vi "get transition voltages.vi"(7 "# of Samples":i32=5, 9 "Enum":enum16{"Ignite", "Quench"}(ring), 10 "Diode":tag, 11 "Main RF":tag) -> (1 "mean":dbl format="%0.2f")   [LabVIEW 2018]
uses:
  <vilib>/DAQmx/write.llb/DAQmx Write (Analog DBL 1Chan 1Samp).vi
  d16da458-7398-4570-a4bb-f738f0a42735.vi
  <vilib>/DAQmx/read.llb/DAQmx Read (Analog DBL 1Chan 1Samp).vi
  <vilib>/DAQmx/create/channels.llb/DAQmx Create Channel (AI-Voltage-Basic).vi
  <vilib>/DAQmx/create/channels.llb/DAQmx Create Channel (AO-Voltage-Basic).vi
  <vilib>/DAQmx/miscellaneous.llb/DAQmx Fill In Error Info.vi
  <vilib>/Analysis/NI_AALBase.lvlib
panel:
  out "Current Diode Voltage":dbl format="%0.2f"
  in  "Slow Factor":dbl=1.0
  out "Threshold":dbl
  out "Waveform Chart":dbl(graph)
  out "Current VO":dbl
  out "Previous Transition Voltage":dbl
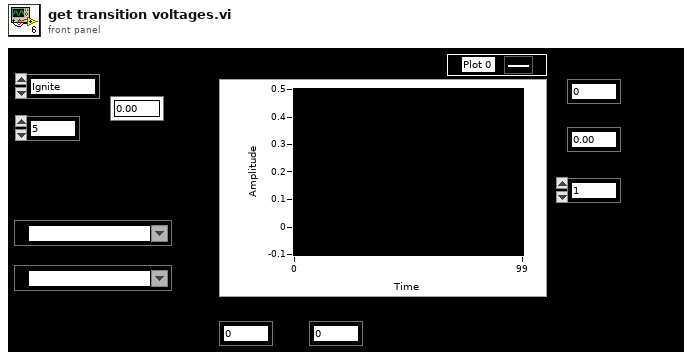
[diagram p1: front panel]
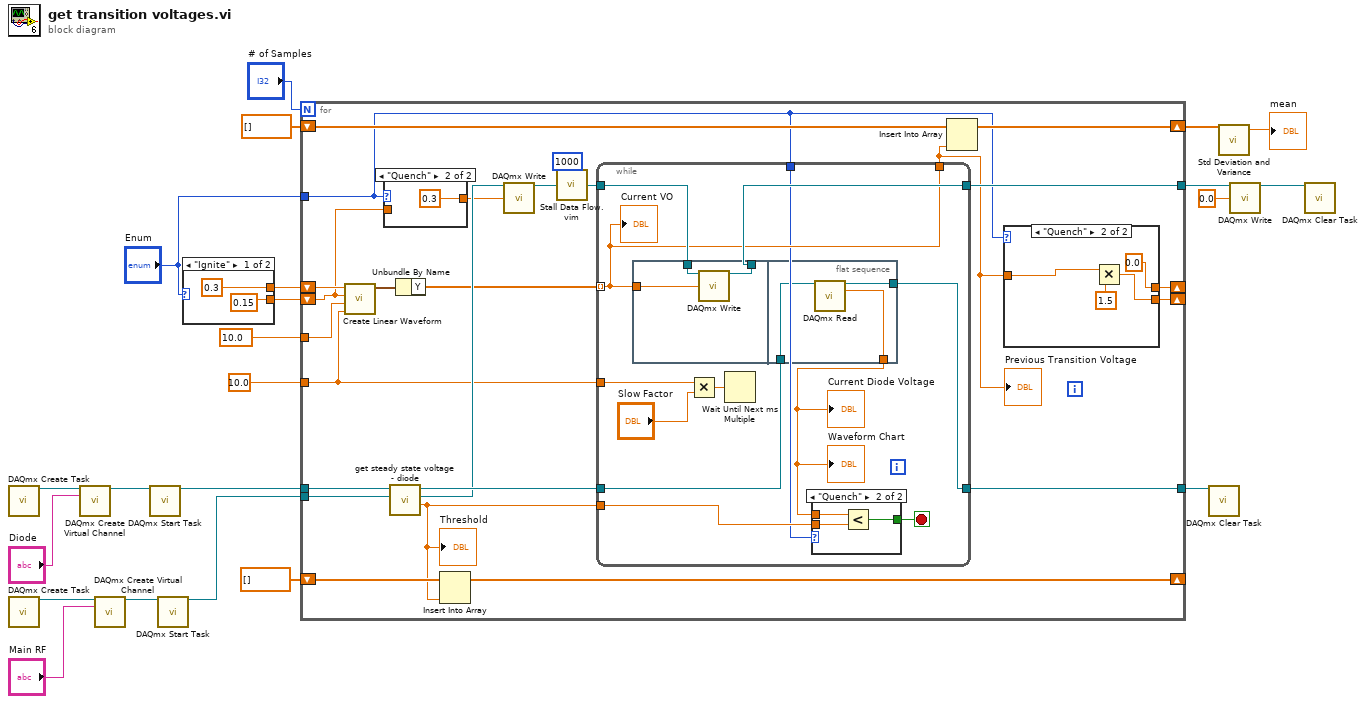
[diagram p0: block diagram]
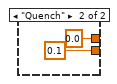
[diagram p2: hidden frame]
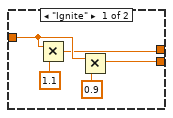
[diagram p3: hidden frame]
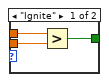
[diagram p5: hidden frame]
diagram:
  n1 = call <vilib>:"DAQmx Create Task.vi"() -> ("task out"=w21:refnum<k21>)  [unwired: 14 in, 1 out]
  n2 = call <vilib>:"DAQmx Create Task.vi"() -> ("task out"=w19:refnum<k21>)  [unwired: 14 in, 1 out]
  n3 = call-poly <vilib>:"DAQmx Create Virtual Channel.vi"("task in"=w21, "physical channels"="Diode") -> ("task out"=w15:refnum<k21>)  [unwired: 12 in, 1 out]
  n4 = call-poly <vilib>:"DAQmx Create Virtual Channel.vi"("task in"=w19, "physical channels"="Main RF") -> ("task out"=w14:refnum<k21>)  [unwired: 12 in, 1 out]
  n5 = call <vilib>:"DAQmx Start Task.vi"("task/channels in"=w15) -> ("task out"=w11:refnum<k21>)  [unwired: 13 in, 1 out]
  n6 = call <vilib>:"DAQmx Start Task.vi"("task/channels in"=w14) -> ("task out"=w10:refnum<k21>)  [unwired: 13 in, 1 out]
  n7 = case shown="\"Ignite\"" "Enum" {
    tunnel: [0.3 ("Vmax") 0.0 ("Vmax")] -> w9
    tunnel: [0.15 ("Vmin") 0.1 ("Vmin")] -> w8
    frame "Ignite" {
    }
    frame "Quench" {
    }
  }
  n8 = for {
    N: "# of Samples" -> [_]
    tunnel: w10 -> [w49]
    tunnel: [w36] -> w17
    tunnel: w11 -> [w50]
    tunnel: 10.0 ("Period") -> [w47]
    tunnel: 10.0 ("dt") -> [w46]
    shift-right: [w35] -> w3
    shift-left: dbl[] [] -> [w34]
    shift-right: [w37] -> _
    shift-left: dbl[] [] -> [w39]
    shift-right: [w33] -> _
    shift-left: w9 -> [w32]
    shift-right: [w28] -> _
    shift-left: w8 -> [w31]
    tunnel: "Enum" -> [w27]
    tunnel: [w30] -> w1
    n9 = call "Create Linear Waveform.vi"("dt"=w46, "Period"=w47, "V Start"=w31, "V End"=w32) -> ("signal out"=w44:waveform(dbl))  [unwired: 7 in]
    n10 = case shown="\"Quench\"" w27 {
      tunnel: [w61 0.3 ("Vmin")] -> w42
      tunnel: w31 -> [w61 _]
      frame "Ignite" {
      }
      frame "Quench" {
      }
    }
    n11 = call "get steady state voltage - diode.vi"("main RF task in"=w49, "Diode Task In"=w50) -> ("Output"=w38:dbl, "Main RF task out"=w48:refnum<k21>, "diode task out"=w51:refnum<k21>)  [unwired: 7 in]
    "Threshold" <- w38
    n12 = Unbundle By Name(w44) -> ("Y"=w43:dbl[])
    n13 = Insert Into Array(array=w39, new element=w38) -> (w37:dbl[])  [unwired: 1 in]
    n14 = call-poly <vilib>:"DAQmx Write.vi"("task/channels in"=w48, "data"=w42) -> ("task out"=w45:refnum<k21>)  [unwired: 11 in, 2 out]
    n15 = call "Stall Data Flow.vim"("value in"=w45, "milliseconds to wait"=u32 1000) -> ("value out"=w41:refnum<k21>)  [unwired: 1 out]
    n16 = while {
      tunnel: w43 -> [w67] mode=indexing
      tunnel: [w74] -> w36
      tunnel: [w67] -> w29
      tunnel: w38 -> [w73]
      tunnel: w51 -> [w66]
      tunnel: w41 -> [w72]
      tunnel: w46 -> [w71]
      tunnel: [w65] -> w30
      tunnel: w27 -> [w63]
      stop <- w69 stop-if-true
      n17 = flat-sequence {
        tunnel: [w83] -> w74
        tunnel: w72 -> [w82]
        tunnel: w67 -> [w81]
        tunnel: w66 -> [w86]
        tunnel: [w85] -> w65
        tunnel: [w84] -> w64
        frame #0 {
          n18 = call-poly <vilib>:"DAQmx Write.vi"("task/channels in"=w82, "data"=w81) -> ("task out"=w83:refnum<k21>)  [unwired: 11 in, 2 out]
        }
        frame #1 {
          n19 = call-poly <vilib>:"DAQmx Read.vi"("task/channels in"=w86) -> ("task out"=w85:refnum<k21>, "data"=w84:dbl)  [unwired: 12 in, 1 out]
        }
      }
      n20 = Multiply(x=w71, y="Slow Factor") -> (x*y=w68:dbl)
      n21 = Wait Until Next ms Multiple(millisecond multiple=w68) -> ()  [unwired: 1 out]
      n22 = case shown="\"Quench\"" w63 {
        tunnel: w73 -> [w77 w80]
        tunnel: [w75 w79] -> w69
        tunnel: w64 -> [w76 w78]
        frame "Ignite" {
          n23 = Greater?(x=w76, y=w77) -> (0:w75:bool)
        }
        frame "Quench" {
          n24 = Less?(x=w78, y=w80) -> (x < y?=w79:bool)
        }
      }
      "Waveform Chart" <- w64
      "Current VO" <- w67
      "Current Diode Voltage" <- w64
    }
    "Previous Transition Voltage" <- w29
    n25 = Insert Into Array(array=w34, new element=w29) -> (w35:dbl[])  [unwired: 1 in]
    n26 = case shown="\"Quench\"" w27 {
      tunnel: [w53 0.0] -> w33
      tunnel: [w52 w59] -> w28
      tunnel: w29 -> [w54 w58]
      frame "Ignite" {
        n27 = Multiply(x=w54, y=1.1) -> (x*y=w53:dbl)
        n28 = Multiply(x=w54, y=0.9) -> (x*y=w52:dbl)
      }
      frame "Quench" {
        n29 = Multiply(x=w58, y=1.5) -> (x*y=w59:dbl)
      }
    }
  }
  n30 = call <vilib>:"DAQmx Clear Task.vi"("task in"=w1) -> ()  [unwired: 14 in, 1 out]
  n31 = call <vilib>:"Std Deviation and Variance.vi"("X"=w3) -> ("mean"=→"mean":dbl)  [unwired: 1 in, 2 out]
  n32 = call-poly <vilib>:"DAQmx Write.vi"("task/channels in"=w17, "data"=0.0) -> ("task out"=w18:refnum<k21>)  [unwired: 11 in, 2 out]
  n33 = call <vilib>:"DAQmx Clear Task.vi"("task in"=w18) -> ()  [unwired: 14 in, 1 out]
